vi "Facade.vi"(0 "Data In":T4, 2 "Display State In":T2, 3 "Container State":T3) -> (6 "Data Out":T4, 7 "Display State Out":T2, 8 "Action":T1)   [LabVIEW 2011, in "Saphirwww.xctl"]
uses:
  <vilib>/_probes/SAPHIR/ViBox - Probes/SaphirwwwButton/Saphirwww.xctl
  <vilib>/_probes/SAPHIR/ViBox - Probes/SaphirwwwButton/Data.ctl
  <vilib>/_xctls/Container State.ctl
  <vilib>/_probes/SAPHIR/ViBox - Probes/SaphirwwwButton/State.ctl
  <vilib>/_xctls/Action.ctl
  <vilib>/Platform/browser.llb/Open URL in Default Browser (string).vi
  <vilib>/_xctls/XControlSupport.lvlib
panel:
  in  "Cluster":cluster{"www":bool}
  # "Provided by"
  # "www.saphir.fr"
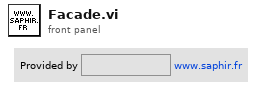
[diagram p1: front panel]
types:
  T1 = typedef "XControlSupport.lvlib/Action.ctl" = cluster{"Data Changed?":bool, "State Changed?":bool, "Action Name":string}
  T2 = typedef "Saphirwww.xctl/State.ctl" = cluster{"CallerViName":string}
  T3 = typedef "XControlSupport.lvlib/Container State.ctl" = cluster{"Indicator?":bool, "Run Mode?":bool, " Refnum":refnum<vi>}
  T4 = typedef "Saphirwww.xctl/Data.ctl" = bool
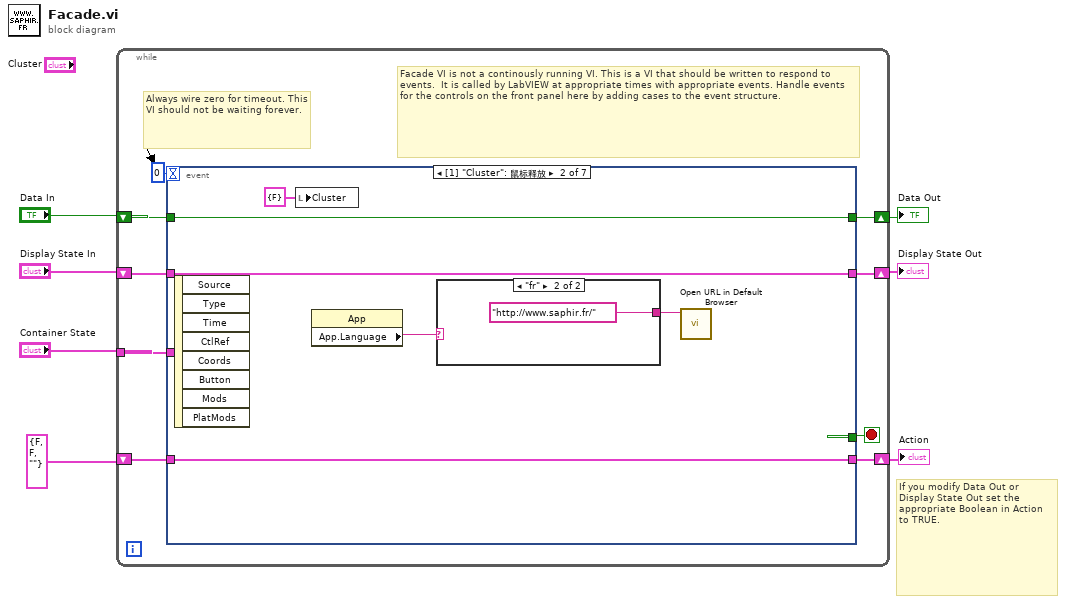
[diagram p0: block diagram]
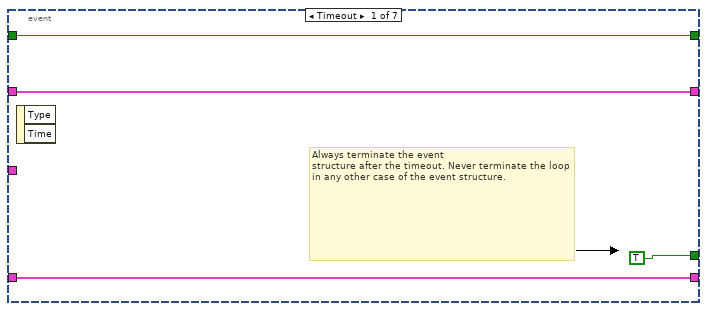
[diagram p2: hidden frame]
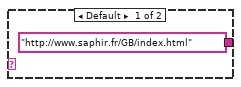
[diagram p3: hidden frame]
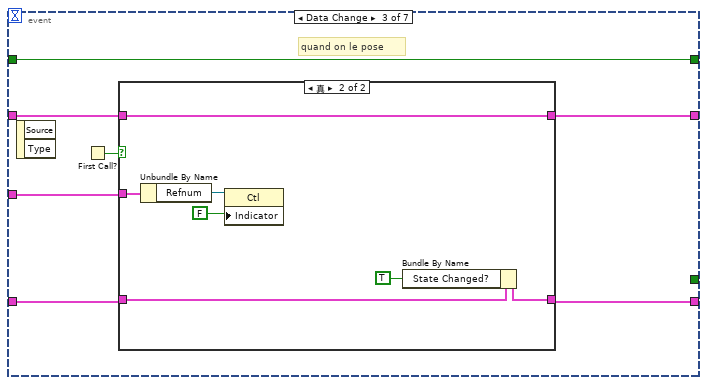
[diagram p4: hidden frame]
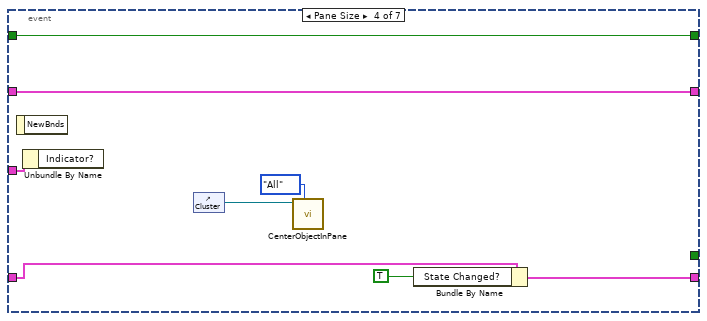
[diagram p6: hidden frame]
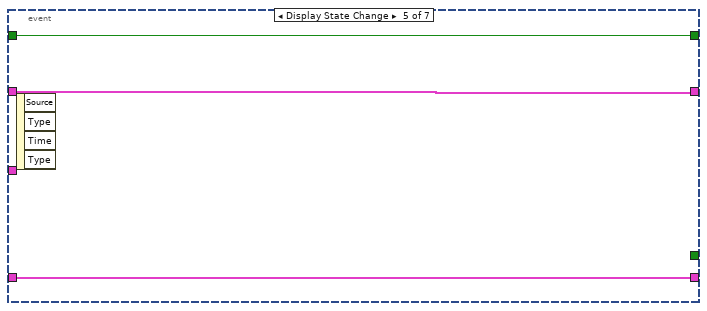
[diagram p7: hidden frame]
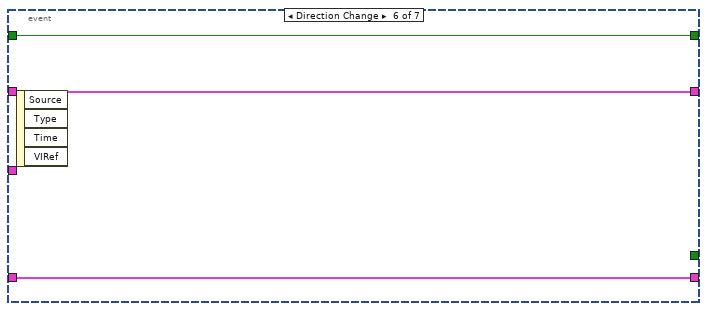
[diagram p8: hidden frame]
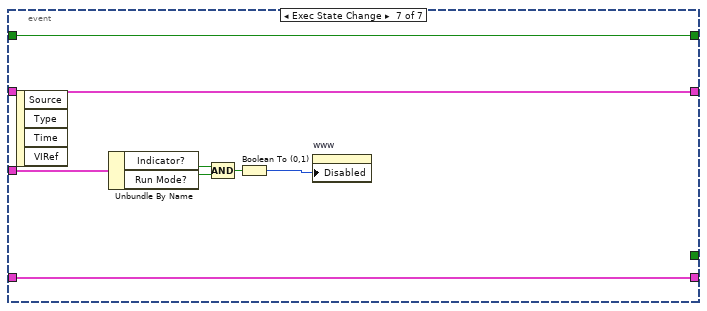
[diagram p9: hidden frame]
diagram:
  # "If you modify Data Out or\nDisplay State Out set the\nappropriate Boolean in Action\nto TRUE."
  n1 = while {
    shift-right: [w16] -> w2
    shift-left: "Display State In" -> [w8]
    tunnel: "Container State" -> [w13]
    shift-right: [w11] -> w3
    shift-left: "Data In" -> [w12]
    shift-right: [w9] -> w1
    shift-left: T1 {"Data Changed?"=FALSE, "State Changed?"=FALSE, "Action Name"=""} ("Action") -> [w10]
    stop <- w15 stop-if-true
    # "Facade VI is not a continously running VI. This is a VI that should be written to respond to events.  It is called by LabVIEW at appropriate times with appropriate events. Handle events for the controls on the front panel here by adding cases to the event structure."
    # "Always wire zero for timeout. This\nVI should not be waiting forever."
    n2 = event shown="[1] \"Cluster\": 鼠标释放" {
      selector: _ -> [_ _ _ _ _ _ _]
      dyn-events: _ -> [_ _ _ _ _ _ _]
      timeout: 0 -> [_ _ _ _ _ _ _]
      tunnel: w8 -> [w18 w25 w32 w50 w54 w58 w59]
      tunnel: [w18 w25 w31 w50 w54 w58 w59] -> w16
      tunnel: [TRUE _ _ _ _ _ _] -> w15
      tunnel: w13 -> [_ _ w34 w52 _ _ w61]
      tunnel: w12 -> [w17 w22 w33 w51 w55 w57 w66]
      tunnel: [w17 w22 w33 w51 w55 w57 w66] -> w11
      tunnel: [w19 w26 w29 w47 w53 w56 w65] -> w9
      tunnel: w10 -> [w19 w26 w30 w49 w53 w56 w65]
      event Timeout {
        # "Always terminate the event\nstructure after the timeout. Never terminate the loop in any other case of the event structure."
        n3 = event-data() -> ()  [unwired: 3 out]
      }
      event "Cluster": Mouse Up {
        n4 = event-data() -> ()  [unwired: 9 out]
        n5 = local write "Cluster"(cluster{"www":bool} {"www"=FALSE} ("Cluster")) -> ()
        n6 = property class="App"() -> ("App.Language"=w21:string)  [unwired: 2 in, 2 out]
        n7 = case shown="\"fr\"" w21 {
          tunnel: ["http://www.saphir.fr/GB/index.html" ("command line") "http://www.saphir.fr/" ("command line")] -> w24
          frame Default {
          }
          frame "fr" {
          }
        }
        n8 = call-poly <vilib>:"Open URL in Default Browser.vi"("URL"=w24) -> ()  [unwired: 1 in, 6 out]
      }
      event Data Change {
        # "quand on le pose"
        n9 = event-data() -> ()  [unwired: 3 out]
        n10 = First Call?() -> (First Call?: T/F=w35:bool)
        n11 = case shown="真" w35 {
          tunnel: w34 -> [_ w44]
          tunnel: w32 -> [w37 w39]
          tunnel: [w37 w39] -> w31
          tunnel: w30 -> [w36 w41]
          tunnel: [w36 w40] -> w29
          frame False {
          }
          frame True {
            n12 = Unbundle By Name(w44) -> ("Refnum"=w43:refnum<vi>)
            n13 = property class="Ctl"(reference=w43, "Indicator"=FALSE) -> ()  [unwired: 1 in, 2 out]
            n14 = Bundle By Name(cluster=w41, "State Changed?"=TRUE) -> (w40:T1)
          }
        }
      }
      event Pane Size {
        n15 = event-data() -> ()  [unwired: 2 out]
        n16 = Unbundle By Name(w52) -> ()  [unwired: 1 out]
        n17 = control-ref of="Cluster"() -> (w45:refnum<vi>)
        n18 = call <vilib>:"CenterObjectInPane.vi"("Mode"=enum16{"All", "Horizontally", "Vertically"}."All", "ObjectToCenterRef"=w45) -> ()  [unwired: 1 in, 9 out]
        n19 = Bundle By Name(cluster=w49, "State Changed?"=TRUE) -> (w47:T1)
      }
      event Display State Change {
        n20 = event-data() -> ()  [unwired: 5 out]
      }
      event Direction Change {
        n21 = event-data() -> ()  [unwired: 5 out]
      }
      event Exec State Change {
        n22 = event-data() -> ()  [unwired: 5 out]
        n23 = Unbundle By Name(w61) -> ("Indicator?"=w62:bool, "Run Mode?"=w64:bool)
        n24 = Compound Arithmetic op=AND(w62, w64) -> (w63:bool)
        n25 = Boolean To (0,1)(Boolean=w63) -> (0, 1=w60:i16)
        n26 = property on="www" class="Bool (严格)"("Disabled"=w60) -> ()  [unwired: 2 in, 2 out]
      }
    }
  }
  "Display State Out" <- w2
  "Data Out" <- w3
  "Action" <- w1
